vi "setHss.vi"(9 "type":T1=enum."Conventional Amp", 11 "index":i32) -> ()   [LabVIEW 2016]
uses:
  <userlib>/atmcd64d.llb/HSSpeed_type typedef.ctl
  variables/imageSettings.vi
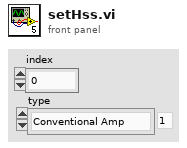
[diagram p1: front panel]
types:
  T1 = typedef "HSSpeed_type typedef.ctl" = enum16{"EM Amp", "Conventional Amp"}
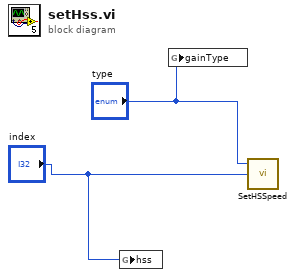
[diagram p0: block diagram]
diagram:
  n1 = global write "imageSettings.vi" "hss"("index") -> ()
  n2 = global write "imageSettings.vi" "gainType"("type") -> ()
  n3 = call <userlib>:"SetHSSpeed.vi"("index"="index", "type"="type") -> ()  [unwired: 2 in, 2 out]
